vi "Input name.vi"() -> (0 "file name":string caption="File name:", 1 "name":string caption="Name:", 2 "valid name":bool)   [LabVIEW 2018]
panel:
  in  "name box":string caption="File name:"
  in  "cancel":bool
  in  "ok":bool
  # "Please enter a name for the new file."
  # "Only leters, numbers, and hyphens are allowed.\nIf the file already exists the configuration will be appended."
  # "Por favor entre o nome do novo arquivo."
  # "Somente letras, números e hífens são permitidos.\nSe o arquivo já existir a configuração será anexada."
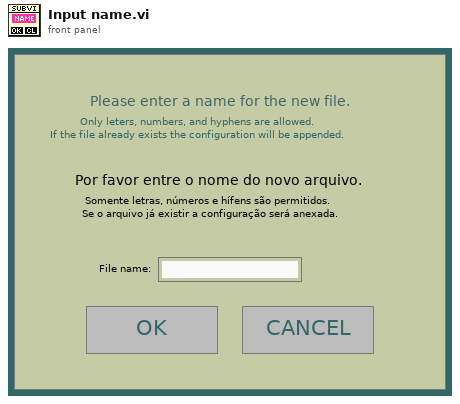
[diagram p1: front panel]
types:
  T1 = enum8{"Enabled", "Disabled", "Disabled and Grayed Out"}
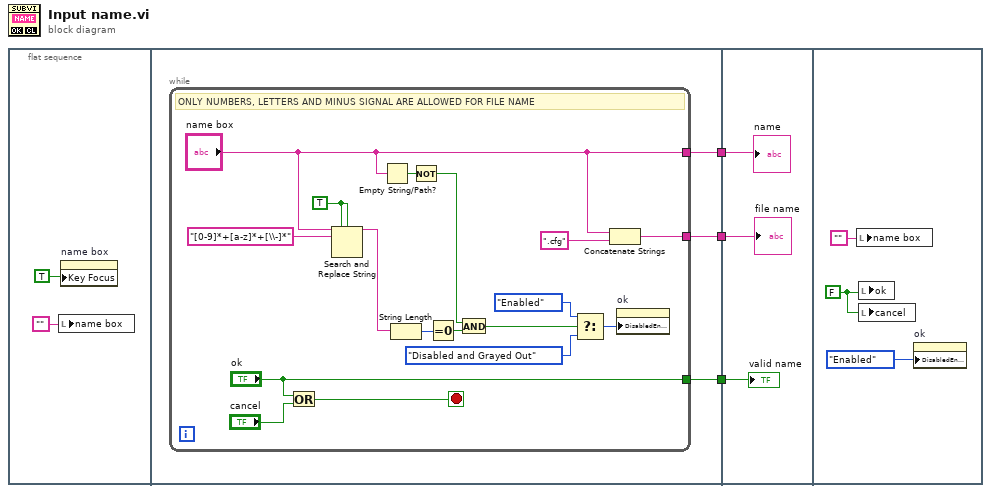
[diagram p0: block diagram]
diagram:
  n1 = flat-sequence {
    tunnel: [w8] -> w3
    tunnel: [w7] -> w2
    tunnel: [w6] -> w1
    tunnel: w3 -> [w27]
    tunnel: w2 -> [w28]
    tunnel: w1 -> [w26]
    frame #0 {
      n2 = local write "name box"("") -> ()
      n3 = property on="name box" class="Str"("Key Focus"=TRUE) -> ()  [unwired: 2 in, 2 out]
    }
    frame #1 {
      n4 = while {
        tunnel: ["name box"] -> w8
        tunnel: ["ok"] -> w7
        tunnel: [w11] -> w6
        stop <- w21 stop-if-true
        w15 = TRUE ("ignore case? (F)")
        # "ONLY NUMBERS, LETTERS AND MINUS SIGNAL ARE ALLOWED FOR FILE NAME"
        n5 = Or(x="ok", y="cancel") -> (x .or. y?=w21:bool)
        n6 = Search and Replace String(replace all?=w15, case sensitive?=w15, input string="name box", search string="[0-9]*+[a-z]*+[\\-]*" ("regular expression")) -> (result string=w12:string)  [unwired: 4 in, 3 out]
        n7 = Empty String/Path?(string/path="name box") -> (empty?=w19:bool)
        n8 = String Length(string=w12) -> (length=w14:i32)
        n9 = Not(x=w19) -> (.not. x?=w18:bool)
        n10 = Equal To 0?(x=w14) -> (x = 0?=w13:bool)
        n11 = And(x=w18, y=w13) -> (x .and. y?=w17:bool)
        n12 = Select(t=T1."Enabled" ("Disabled"), s=w17, f=T1."Disabled and Grayed Out" ("Disabled")) -> (s? t:f=w23:T1)
        n13 = Concatenate Strings("name box", ".cfg" ("string")) -> (w11:string)
        n14 = property on="ok" class="Bool (strict)"("DisabledEnum"=w23) -> ()  [unwired: 2 in, 2 out]
      }
    }
    frame #2 {
      "name" <- w27
      "valid name" <- w28
      "file name" <- w26
    }
    frame #3 {
      w30 = FALSE
      n15 = local write "name box"("") -> ()
      n16 = local write "ok"(w30) -> ()
      n17 = local write "cancel"(w30) -> ()
      n18 = property on="ok" class="Bool (strict)"("DisabledEnum"=T1."Enabled" ("Disabled")) -> ()  [unwired: 2 in, 2 out]
    }
  }
